vi "SetBoundsBySocket.vi"(8 "Error In":errorcluster, 9 "Test Name":string, 10 "Test Socket":i32, 11 "vi reference":refnum<vi>) -> (0 "Error Out":errorcluster)   [LabVIEW 2011]
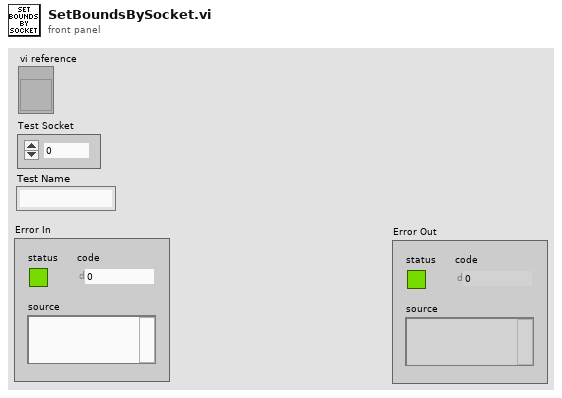
[diagram p1: front panel]
types:
  T1 = typedef "LVRectTypeDef.ctl" = cluster{"left":i16, "top":i16, "right":i16, "bottom":i16}
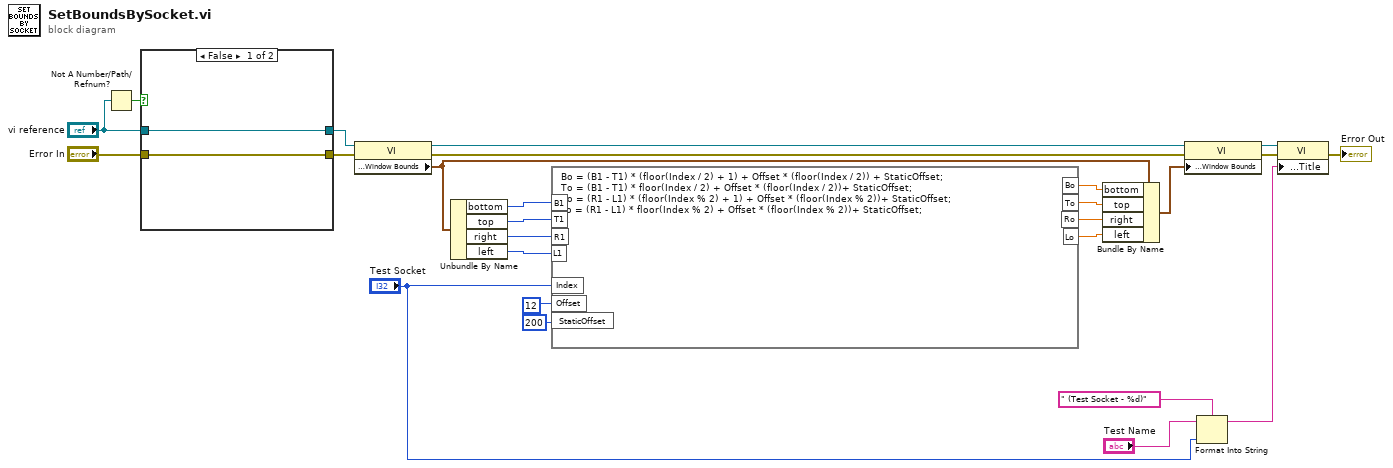
[diagram p0: block diagram]
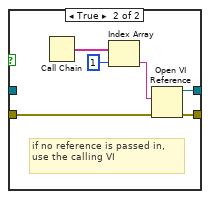
[diagram p2: hidden frame]
diagram:
  n1 = Not A Number/Path/Refnum?(number/path/refnum="vi reference") -> (NaN/Path/Refnum?=w3:bool)
  n2 = case shown="False" w3 {
    tunnel: [w28 w32] -> w25
    tunnel: [w27 w31] -> w20
    tunnel: "vi reference" -> [w28 _]
    tunnel: "Error In" -> [w27 w29]
    frame False {
    }
    frame True {
      # "if no reference is passed in, use the calling VI"
      n3 = Call Chain() -> (call chain=w34:string[])
      n4 = Index Array(array=w34, index=1) -> (element=w33:string)
      n5 = Open VI Reference(vi path=w33, error in (no error)=w29) -> (vi reference=w32:refnum<vi>, error out=w31:errorcluster)  [unwired: 4 in]
    }
  }
  n6 = property class="VI"(reference=w25, error in=w20) -> (reference out=w26:refnum<vi>, error out=w19:errorcluster, "Front Panel Window:Window Bounds"=w11:T1)
  n7 = Unbundle By Name(w11) -> ("bottom"=w16:i16, "top"=w15:i16, "right"=w14:i16, "left"=w13:i16)
  n8 = formula code="Bo = (B1 - T1) * (floor(Index / 2) + 1) + Offset * (floor(Index / 2)) + StaticOffset;\nTo = (B1 - T1) * floor(Index / 2) + Offset * (floor(Index / 2))+ StaticOffset;\nRo = (R1 - L1) * (floor(Index % 2) + 1) + Offset * (floor(Index % 2))+ StaticOffset;\nLo = (R1 - L1) * floor(Index % 2) + Offset * (floor(Index % 2))+ StaticOffset;"("B1"=w16, "T1"=w15, "R1"=w14, "L1"=w13, "Index"="Test Socket", "Offset"=12, "StaticOffset"=200) -> ("Bo"=w10:dbl, "To"=w9:dbl, "Ro"=w8:dbl, "Lo"=w7:dbl)
  n9 = Bundle By Name(cluster=w11, "bottom"=w10, "top"=w9, "right"=w8, "left"=w7) -> (w12:T1)
  n10 = property class="VI"(reference=w26, error in=w19, "Front Panel Window:Window Bounds"=w12) -> (reference out=w24:refnum<vi>, error out=w18:errorcluster)
  n11 = Format Into String(format string=" (Test Socket - %d)", initial string="Test Name", "Test Socket") -> (resulting string=w21:string)  [unwired: 1 in, 1 out]
  n12 = property class="VI"(reference=w24, error in=w18, "Front Panel.Title"=w21) -> (error out=→"Error Out":errorcluster)  [unwired: 1 out]
